vi "Global_variables.vi"() -> ()   [LabVIEW 2018]
panel:
  in  "pos_init":dbl
  in  "mid_encoder":dbl
  in  "Enter_RUN_Flag":dbl
  in  "TEST_A_PWM":dbl
  in  "TEST_P_PWM":dbl
  in  "way_turn":dbl
  in  "state":dbl
  in  "zhongzhi":dbl=3085.0
  in  "Flag_Postion":dbl
  in  "Count_Position":dbl
  in  "Ratio":dbl
  in  "Count_qb":dbl
  in  "Flag_qb 2":dbl
  in  "Flag_Target":dbl
  in  "Count_Moto":dbl
  in  "Moto_qb":dbl
  in  "Position_PWM":dbl
  in  "Balance_PWM":dbl
  in  "Count_P2":dbl
  in  "Flag_qb":dbl
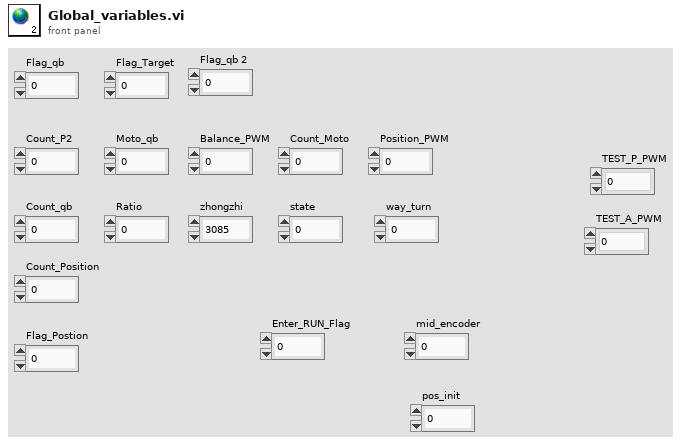
[diagram p1: front panel]
diagram:
